vi "createStopEvent.vi"(8 "error in (no error)":errorcluster) -> (0 "error out":errorcluster, 2 "stopEventRef":refnum<user-event>, 3 "eventRegRef":refnum<event-registration>)   [LabVIEW 2017, in "User Event - Stop.lvlib"]
doc: "Create a boolean user event that will be used to stop the event loop from the message handling loop."
uses:
  User Event - Stop.lvlib
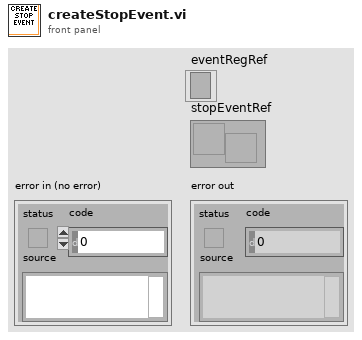
[diagram p1: front panel]
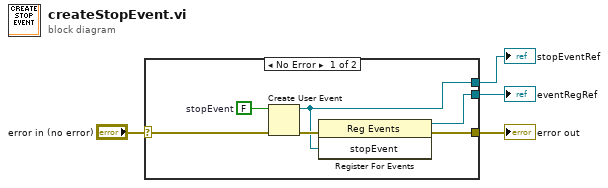
[diagram p0: block diagram]
diagram:
  n1 = case shown="No Error" "error in (no error)" {
    selector: "error in (no error)" -> [w9 w11]
    tunnel: [w6 _] -> w1
    tunnel: [w7 w11] -> w4
    tunnel: [w5 _] -> w2
    frame No Error {
      w10 = FALSE  # stopEvent
      n2 = Create User Event(user event datatype=w10, error in=w9) -> (user event=w6:refnum<user-event>, error out=w8:errorcluster)
      n3 = register-events(error in=w8, w6) -> (reference out=w5:refnum<event-registration>, error out=w7:errorcluster)  [unwired: 1 in]
    }
    frame Error {
    }
  }
  "error out" <- w4
  "eventRegRef" <- w2
  "stopEventRef" <- w1
